vi "V - prędkość postępowa.vi"() -> ()   [LabVIEW 2015, in "Biblioteka moduł map v3.lvlib" / "Zmienne.lvlib"]
uses:
  Zmienne.lvlib
panel:
  in  "V - prędkość postępowa":dbl
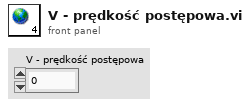
[diagram p1: front panel]
diagram:
